vi "oa_Multistage Interpolation Filter.vi"(7 "reset? (True)":bool=TRUE, 8 "error in (no error)":errorcluster, 9 "interpolation filters":T1[](array[typedef]) {"coefficients" format="%.2f"}, 11 "x[n]":dbl[](array[numeric]) format="%.2f") -> (0 "error out":errorcluster, 3 "x[n] out":dbl[](array[numeric]) format="%.2f")   [LabVIEW 2017, in "SoundVib_Resampling.lvlib"]
uses:
  <vilib>/addons/Sound and Vibration/Order Analysis/Resample Order Tracking/SoundVib_Resampling.lvlib
  <vilib>/addons/_NISVFA/_Shared subVIs/Controls/OAT Decimation Filter.ctl
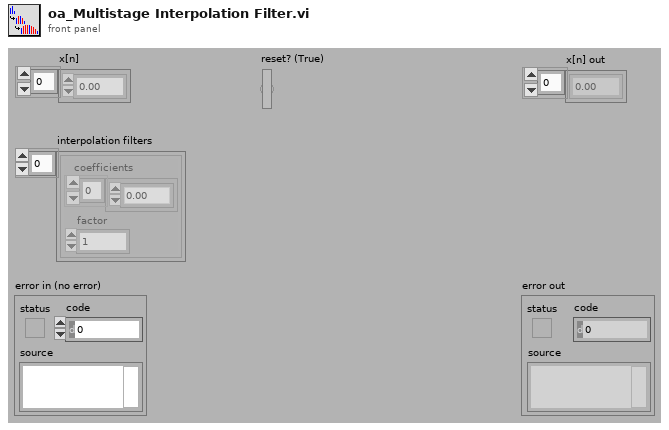
[diagram p1: front panel]
types:
  T1 = typedef "OAT Decimation Filter.ctl" = cluster{"coefficients":dbl[], "factor":i32}
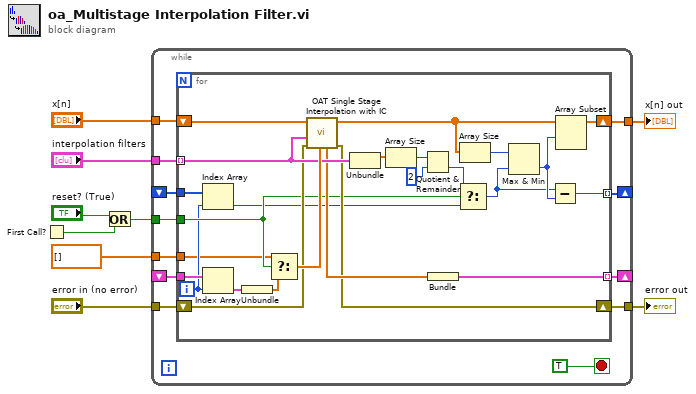
[diagram p0: block diagram]
diagram:
  n1 = First Call?() -> (First Call?: T/F=w8:bool)
  n2 = Or(x="reset? (True)", y=w8) -> (x .or. y?=w4:bool)
  n3 = while {
    shift-right: [w15] -> _
    shift-left: _ -> [w14]
    tunnel: "x[n]" -> [w21]
    tunnel: "interpolation filters" -> [w20]
    tunnel: "error in (no error)" -> [w19]
    tunnel: [w18] -> w5
    tunnel: w4 -> [w16]
    tunnel: [w13] -> w2
    shift-right: [w12] -> _
    shift-left: _ -> [w11]
    tunnel: dbl[] [] ("t") -> [w10]
    stop <- TRUE stop-if-true
    n4 = for {
      shift-right: [w39] -> w13
      shift-left: w21 -> [w45]
      tunnel: w20 -> [w44] mode=indexing
      shift-right: [w38] -> w18
      shift-left: w19 -> [w37]
      tunnel: w16 -> [w28]
      tunnel: [w42] -> w15 mode=indexing
      tunnel: w14 -> [w41]
      tunnel: [w29] -> w12 mode=indexing
      tunnel: w11 -> [w24]
      tunnel: w10 -> [w22]
      i -> [w25]
      n5 = Index Array(array=w24, index=w25) -> (element=w23:i32)
      n6 = Index Array(array=w41, index=w25) -> (element=w40:cluster{"final state":dbl[]})
      n7 = Unbundle(w40) -> ("final state"=w36:dbl[])
      n8 = Select(t=w22, s=w28, f=w36) -> (s? t:f=w46:dbl[])
      n9 = call <vilib>:"OAT Single Stage Interpolation with IC.vi"("initial state"=w46, "error in (no error)"=w37, "filter"=w44, "X"=w45) -> ("error out"=w38:errorcluster, "Y"=w32:dbl[], "final state"=w43:dbl[])  [unwired: 5 in]
      n10 = Unbundle(w44) -> ("coefficients"=w35:dbl[])  [unwired: 1 out]
      n11 = Array Size(array=w35) -> (size(s)=w34:i32)
      n12 = Quotient & Remainder(x=w34, y=2) -> (floor(x/y)=w27:i32)  [unwired: 1 out]
      n13 = Bundle("final state"=w43) -> (w42:cluster{"final state":dbl[]})  [unwired: 1 in]
      n14 = Select(t=w27, s=w28, f=w23) -> (s? t:f=w26:i32)
      n15 = Array Size(array=w32) -> (size(s)=w31:i32)
      n16 = Max & Min(x=w31, y=w26) -> (min(x,y)=w30:i32)  [unwired: 1 out]
      n17 = Subtract(x=w26, y=w30) -> (x-y=w29:i32)
      n18 = Array Subset(array=w32, index=w30) -> (w39:dbl[])  [unwired: 1 in]
    }
  }
  "error out" <- w5
  "x[n] out" <- w2
